vi "WaveTank.vi"() -> ()   [LabVIEW 2025]
uses:
  install/bin/libwavetanktestinglib.dll
panel:
  out "ErrMsg":string
  out "RootName":string
  in  "WT_InputFile":string="..\\..\\python\\wavetankconfig.in"
  out "path":path
  out "Application Directory":path
  out "ErrStat":i32
  in  "Testing in":errorcluster
  out "Testing Out":errorcluster
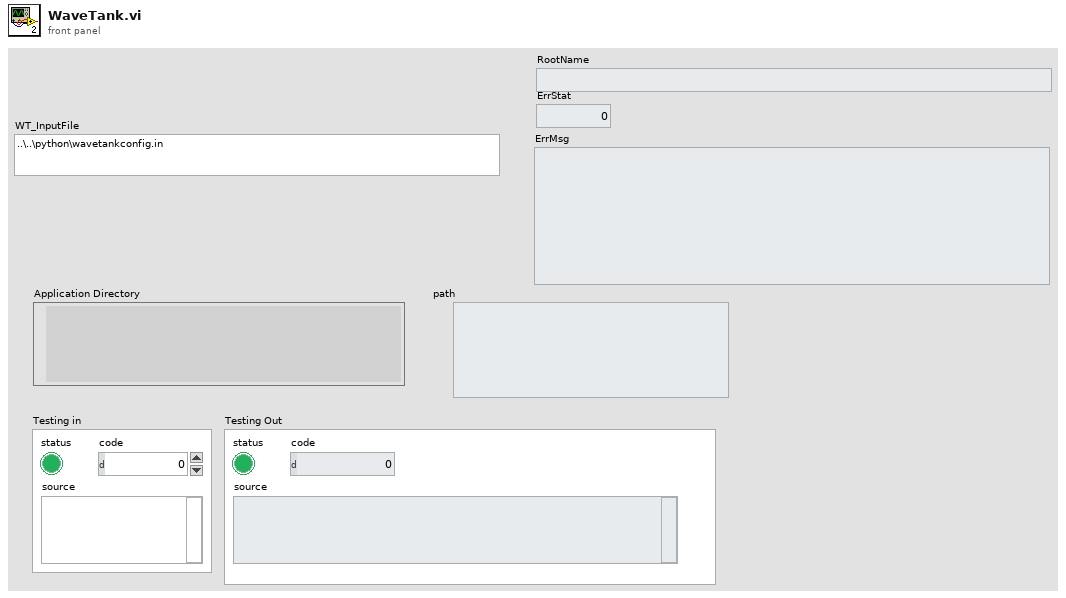
[diagram p1: front panel]
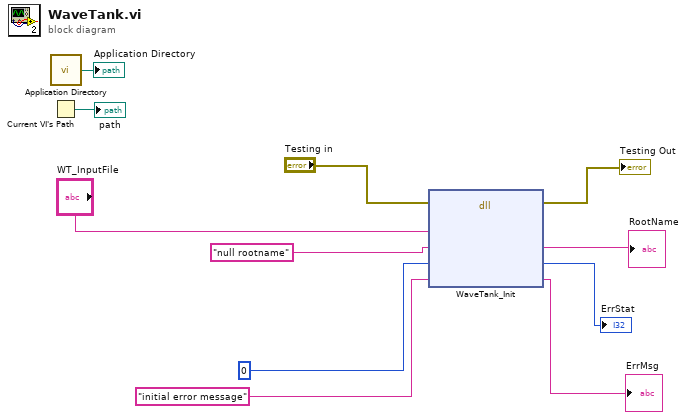
[diagram p0: block diagram]
diagram:
  n1 = call <vilib>:"Application Directory.vi"() -> ("Application Directory"=→"Application Directory":path)
  n2 = Current VI's Path() -> (path=→"path":path)
  n3 = dll-call lib="C:/Users/aplatt/Documents/software-development/GitHub/openfast/install/bin/libwavetanktestinglib.dll" fn="WaveTank_Init"(error in="Testing in", "WT_InputFile_C"="WT_InputFile", "RootName_C"="null rootname", "ErrStat_C"=0, "ErrMsg_C"="initial error message") -> (error out=→"Testing Out":errorcluster, "RootName_C"=→"RootName":string, "ErrStat_C"=→"ErrStat":i32, "ErrMsg_C"=→"ErrMsg":string)  [unwired: 4 in, 1 out]
